vi "TotalAlkalinityTool.vi"() -> ()   [LabVIEW 2010]
uses:
  Misc/HCl_volume_global.vi
panel:
  out "In hold?":bool
  out "Hold Start Time":timestamp
  in  "Tab Control":T1(tab)
  out "Cell Temp (dup)":dbl
  out "Initialized?":bool
  in  "Initialize Instruments":bool
  in  "Run Settings":T2={"Operator"="", "Sample (or CRM) ID"="", "Sample Temp"=0.0, "Salinity"=0.0, "Sample Units"=FALSE, "Sample Size"=0.0, "Operation Mode"=TRUE}
  in  "Data Directory":path
  in  "stop":bool
  in  "Begin Titration":bool
  in  "Configuration":T3={"Alkalinity Calculation Functions"={"HCl Temp Correction Function"="", "Sample Temp Correction Function"="", "Dosimat Correction Function"="", "Cell Temp Correction Function"="", "HCl Density Function"=""}, "Instrument Settings"={"Relay Port"="COM6", "Agilent Port"="COM5", "Dosimat Port"="COM4", "Thermal Coeffients Path"=path ""}, "Titration Settings"={"Hold Time (sec)"=300, "Initial HCl Increment"=0.0, "Target EMF"=0.0, "Agilent Monitoring Refresh Period"=0.0, "Small HCl Increment"=0.0, "Number of Titration Points"=0}, "Other Settings"={"HCl Concentration"=0.0, "HCl Lot ID"=""}, "Electrode Settings"={"Probe ID - Electrode 1 "=0, "Channel - Electrode 1"=0, "Probe ID - Electrode 2"=0, "Channel - Electrode 2"=0}} {"Electrode Settings"."Probe ID - Electrode 2" items=["OLD1", "OLD2", "OV1-106509", "OW1-10628", "OW1-10659"]; "Electrode Settings"."Probe ID - Electrode 1" items=["OLD1", "OLD2", "OV1-106509", "OW1-10628", "OW1-10659"]}
  in  "Save Config":bool
  out "Voltage 2":dbl
  out "Voltage 1":dbl
  out "Titration Pts Left":dbl
  out "Electrode 2 Results":T4 {"k" format="%.5g"; "Final E0" format="%#.5g"; "mse" format="%.2g"}
  out "Electrode 1 Results":T4 {"k" format="%.5g"; "Final E0" format="%#.5g"; "mse" format="%#_3g"}
  out "Titration State":string
  out "Titrating?":bool
  out "Titration EMFs":cluster{"x values":dbl[], "voltages":dbl[]}[](graph)
  out "Voltage Standard Deviation":T5(graph)
  out "Hold Time Remaining":dbl
  out "Burette Temp 2":dbl
  out "Cell Temp":dbl
  out "Acid Temp":dbl
  out "Burette Temp 1":dbl
  out "Room Temp":dbl
  out "HCl Volume (Uncorr)":dbl
  in  "Probe to Follow":bool
  out "E0 Values":cluster{timestamp[], dbl[]}[](graph)
  out "Alakalinity Variance From References":cluster{timestamp[], dbl[]}[](graph)
  in  "Load QC Data":bool
  out "File Error Out":errorcluster
  # "It is important that these settings be correctly set for each run."
  # "y = -0.0003x2 + 1.0021x - 0.003"
  # "Required Inputs"
  # "It is imortant that these settings be correctly set for each run."
  # "These configuration settings are stored in an XML file and can be updated for a specific run and then discarded, but can also be saved by clicking the button to the right.\n\nIf you need to change the instrument port settings, run the config_file_accessor vi in the Misc directory. That iwll let you create a new configuration set."
  # "add new electrode using qc_data_accessor"
  # "This control only works when titration is not actively taking place"
  # "Titration Results"
  # "Temps"
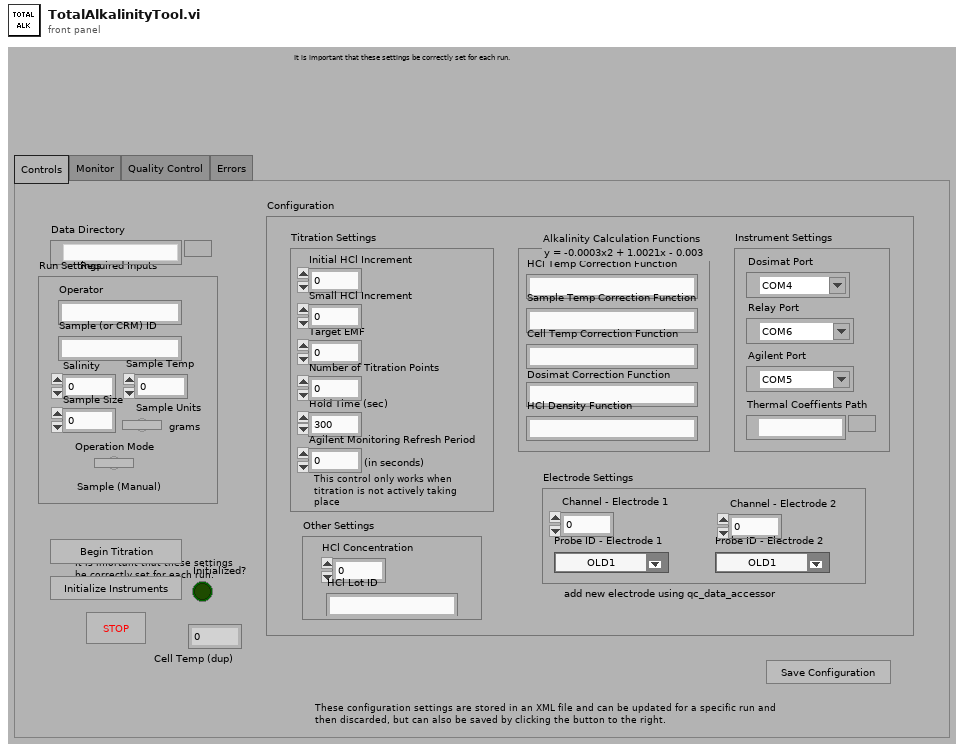
[diagram p1: front panel]
types:
  T1 = enum32{"Controls", "Monitor", "Quality Control", "Errors"}
  T2 = cluster{"Operator":string, "Sample (or CRM) ID":string, "Sample Temp":dbl, "Salinity":dbl, "Sample Units":bool, "Sample Size":dbl, "Operation Mode":bool}
  T3 = cluster{"Alkalinity Calculation Functions":cluster{"HCl Temp Correction Function":string, "Sample Temp Correction Function":string, "Dosimat Correction Function":string, "Cell Temp Correction Function":string, "HCl Density Function":string}, "Instrument Settings":cluster{"Relay Port":refnum<visa-resource-name>, "Agilent Port":refnum<visa-resource-name>, "Dosimat Port":refnum<visa-resource-name>, "Thermal Coeffients Path":path}, "Titration Settings":cluster{"Hold Time (sec)":i16, "Initial HCl Increment":dbl, "Target EMF":dbl, "Agilent Monitoring Refresh Period":dbl, "Small HCl Increment":dbl, "Number of Titration Points":i32}, "Other Settings":cluster{"HCl Concentration":dbl, "HCl Lot ID":string}, "Electrode Settings":cluster{"Probe ID - Electrode 1 ":u16, "Channel - Electrode 1":i32, "Probe ID - Electrode 2":u16, "Channel - Electrode 2":i32}}
  T4 = cluster{"Total Alkalinity":dbl, "mse":dbl, "Final E0":dbl, "k":dbl}
  T5 = cluster{"x values":dbl[], "voltage stddevs":dbl[]}[]
  T6 = cluster{"Time Stamp":timestamp, "Titration Stage":string, "Average Voltage":dbl, "Burette Temp Average":dbl, "Voltage 1":dbl, "Voltage 2":dbl, "Voltage 1 StandDev":dbl, "Voltage 2 StandDev":dbl, "Burette Temp 1":dbl, "Burette Temp 2":dbl, "Cell Temp":dbl, "Acid Temp":dbl, "Room Temp":dbl}[]
  T7 = typedef "LVStringsAndValuesArrayTypeDef.ctl" = cluster{"String":string, "Value":ext}[]
  T8 = cluster{"VISA resource out":refnum<visa-resource-name>, "error out":errorcluster}
  T9 = cluster{"Dosimat Port out":refnum<visa-resource-name>, "Error out":errorcluster}
  T10 = cluster{"Data Flag":string, "Notes":string, "Probe 1 Results":cluster{"Total Alkalinity":dbl, "mse":dbl, "Final E0":dbl, "k":dbl}, "Probe 2 Results":cluster{"Total Alkalinity":dbl, "mse":dbl, "Final E0":dbl, "k":dbl}}
  T11 = cluster{"HCl Temp Correction Function":string, "Sample Temp Correction Function":string, "Dosimat Correction Function":string, "Cell Temp Correction Function":string, "HCl Density Function":string}
  T12 = cluster{"Hold Time (sec)":i16, "Initial HCl Increment":dbl, "Target EMF":dbl, "Agilent Monitoring Refresh Period":dbl, "Small HCl Increment":dbl, "Number of Titration Points":i32}
  T13 = cluster{"HCl Concentration":dbl, "HCl Lot ID":string}
  T14 = cluster{"Relay Port":refnum<visa-resource-name>, "Agilent Port":refnum<visa-resource-name>, "Dosimat Port":refnum<visa-resource-name>, "Thermal Coeffients Path":path}
  T15 = cluster{"Probe ID - Electrode 1 ":u16, "Channel - Electrode 1":i32, "Probe ID - Electrode 2":u16, "Channel - Electrode 2":i32}
  T16 = cluster{"Time":timestamp, "Operator":string, "Flag":string, "CRM ID":string, "HCl Batch ID":string, "CRM Certified Alk":dbl, "Salinity":dbl, "HCl Temp (uncorr)":dbl, "Cell Temp Mean (uncorr)":dbl, "Measured Alk":dbl, "MSE":dbl, "Final E0":dbl, "k":dbl}[]
  T17 = cluster{"Time":timestamp, "Operator":string, "Flag":string, "CRM ID":string, "HCl Batch ID":string, "CRM Certified Alk":dbl, "Salinity":dbl, "HCl Temp (uncorr)":dbl, "Cell Temp Mean (uncorr)":dbl, "Measured Alk":dbl, "MSE":dbl, "Final E0":dbl, "k":dbl}[][]
  T18 = cluster{"Time Stamp":timestamp, "Titration Stage":string, "Average Voltage":dbl, "Burette Temp Average":dbl, "Voltage 1":dbl, "Voltage 2":dbl, "Voltage 1 StandDev":dbl, "Voltage 2 StandDev":dbl, "Burette Temp 1":dbl, "Burette Temp 2":dbl, "Cell Temp":dbl, "Acid Temp":dbl, "Room Temp":dbl}
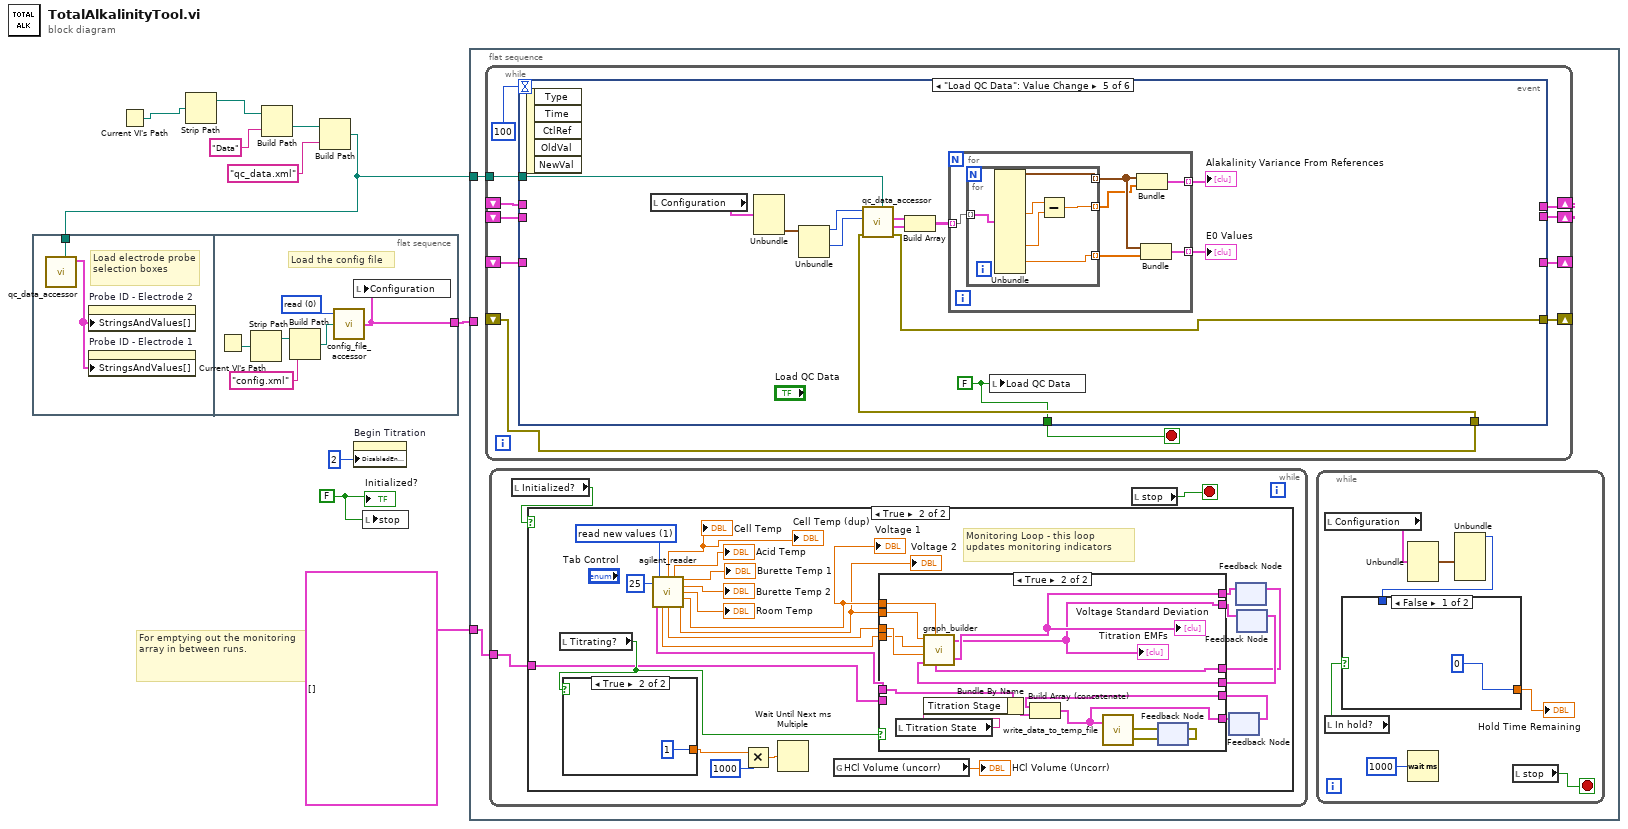
[diagram p0: block diagram]
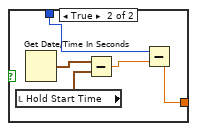
[diagram p2: hidden frame]
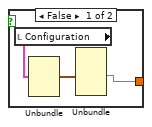
[diagram p4: hidden frame]
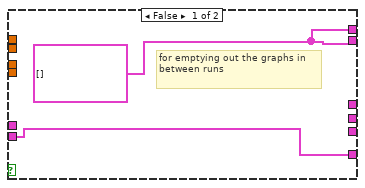
[diagram p5: hidden frame]
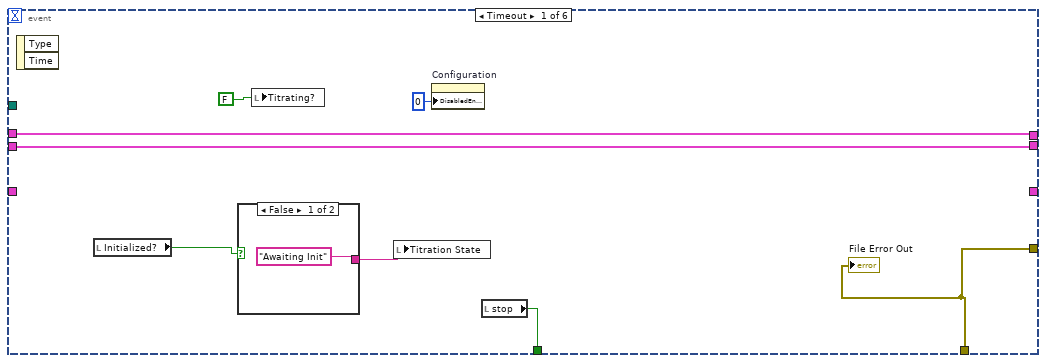
[diagram p6: hidden frame]
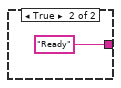
[diagram p7: hidden frame]
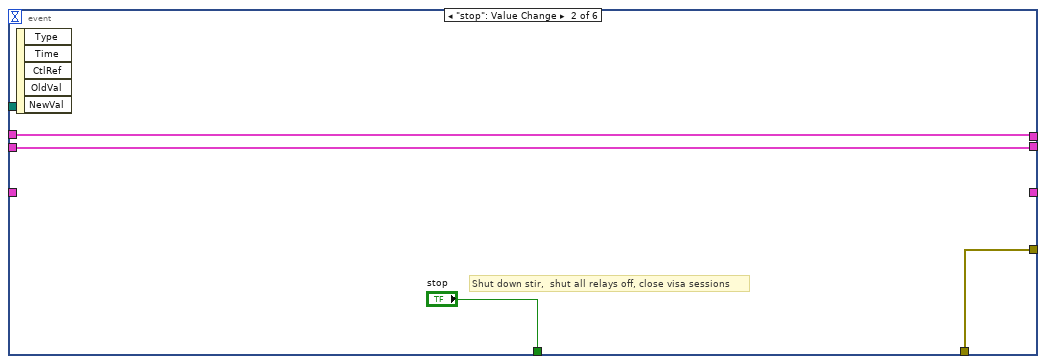
[diagram p8: hidden frame]
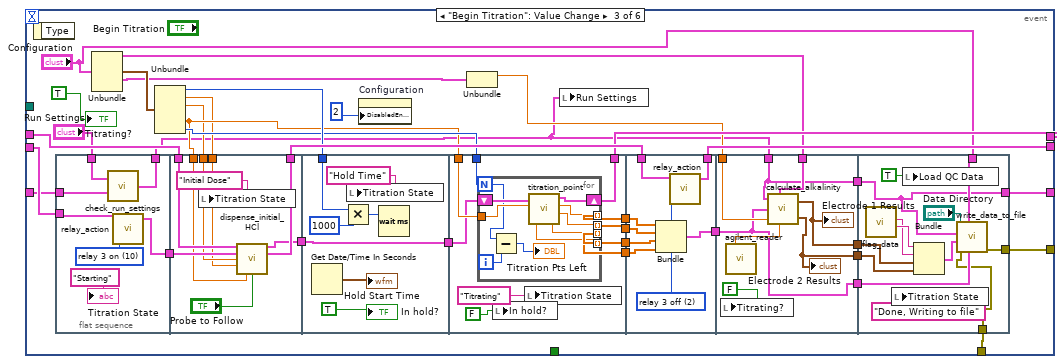
[diagram p9: hidden frame]
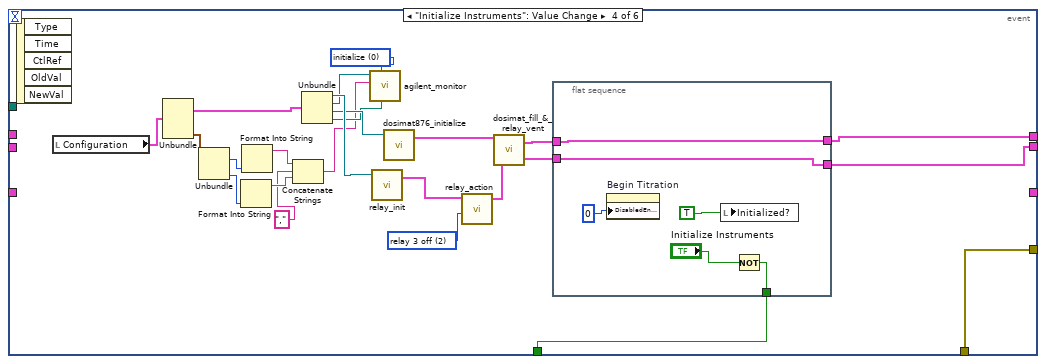
[diagram p10: hidden frame]
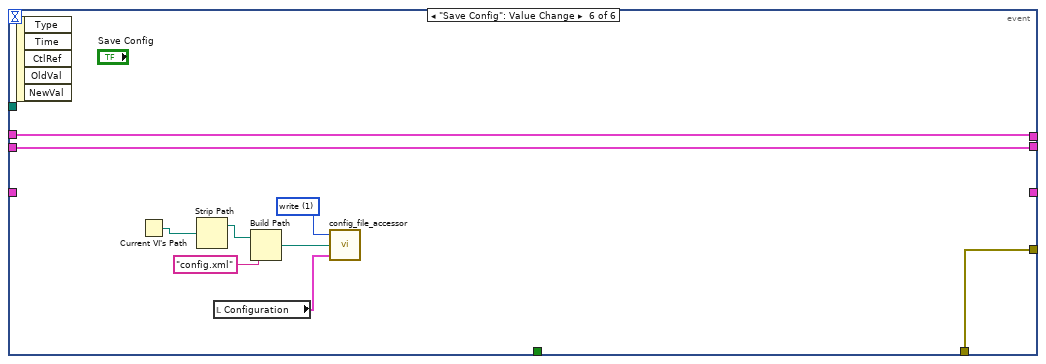
[diagram p11: hidden frame]
diagram:
  w7 = FALSE
  # "For emptying out the monitoring array in between runs."
  n1 = flat-sequence {
    tunnel: w1 -> [w11]
    tunnel: [w13] -> w8
    frame #0 {
      # "Load electrode probe selection boxes"
      n2 = call "qc_data_accessor.vi"("Path"=w11) -> ("Electrode Selection Options"=w12:T7)  [unwired: 7 in, 3 out]
      n3 = property on="Probe ID - Electrode 2" class="Ring (strict)"("StringsAndValues[]"=w12) -> ()  [unwired: 2 in, 2 out]
      n4 = property on="Probe ID - Electrode 1" class="Ring (strict)"("StringsAndValues[]"=w12) -> ()  [unwired: 2 in, 2 out]
    }
    frame #1 {
      w16 = u8 0 items=["read", "write"] ("Action")
      # "Load the config file"
      n5 = Current VI's Path() -> (path=w15:path)
      n6 = Strip Path(path=w15) -> (stripped path=w14:path)  [unwired: 1 out]
      n7 = Build Path(base path=w14, name or relative path="config.xml") -> (appended path=w17:path)
      n8 = call "config_file_accessor.vi"("File Path"=w17, "Action"=w16) -> ("Configuration Out"=w13:T3)  [unwired: 1 in]
      n9 = local write "Configuration"(w13) -> ()
    }
  }
  n10 = Current VI's Path() -> (path=w3:path)
  n11 = Strip Path(path=w3) -> (stripped path=w2:path)  [unwired: 1 out]
  n12 = Build Path(base path=w2, name or relative path="Data") -> (appended path=w4:path)
  n13 = Build Path(base path=w4, name or relative path="qc_data.xml") -> (appended path=w1:path)
  n14 = property on="Begin Titration" class="Bool"("DisabledEnum"=2) -> ()  [unwired: 2 in, 2 out]
  n15 = local write "stop"(w7) -> ()
  n16 = flat-sequence {
    tunnel: T6 [] ("Data Array") -> [w20]
    tunnel: w8 -> [_]
    tunnel: w1 -> [w19]
    frame #0 {
      n17 = while {
        shift-right: [w89] -> _
        shift-left: _ -> [w90]
        shift-right: [w88] -> _
        shift-left: _ -> [w91]
        shift-right: [w86] -> _
        shift-left: _ -> [w85]
        shift-right: [w84] -> _
        shift-left: _ -> [w83]
        tunnel: w19 -> [w82]
        stop <- w92 stop-if-true
        n18 = event shown="[4] \"Load QC Data\": Value Change" {
          selector: _ -> [_ _ _ _ _ _]
          dyn-events: _ -> [_ _ _ _ _ _]
          timeout: 100 -> [_ _ _ _ _ _]
          tunnel: [w93 "stop" _ w237 w247 _] -> w92
          tunnel: w91 -> [w98 w104 w141 _ _ w272]
          tunnel: w90 -> [w99 w105 w140 _ _ w273]
          tunnel: [w99 w105 w136 w225 _ w273] -> w89
          tunnel: [w98 w104 w135 w224 _ w272] -> w88
          tunnel: [w94 w103 w112 w214 w248 w269] -> w86
          tunnel: w85 -> [w94 w103 w111 w214 w249 w269]
          tunnel: [_ _ w110 _ _ _] -> w84
          tunnel: w83 -> [_ _ w108 _ _ _]
          tunnel: w82 -> [_ _ _ _ w244 _]
          event Timeout {
            n19 = event-data() -> ()  [unwired: 1 in, 2 out]
            n20 = local read "Initialized?"() -> (w95:bool)
            n21 = case shown="False" w95 {
              tunnel: ["Awaiting Init" "Ready"] -> w100
              frame False {
              }
              frame True {
              }
            }
            n22 = local write "Titrating?"(FALSE) -> ()
            n23 = local write "Titration State"(w100) -> ()
            n24 = property on="Configuration" class="Clust (strict)"("DisabledEnum"=0) -> ()  [unwired: 2 in, 2 out]
            n25 = local read "stop"() -> (w93:bool)
            "File Error Out" <- w94
          }
          event "stop": Value Change {
            # "Shut down stir,  shut all relays off, close visa sessions"
            n26 = event-data() -> ()  [unwired: 1 in, 5 out]
          }
          event "Begin Titration": Value Change {
            n27 = event-data() -> ()  [unwired: 1 in, 1 out]
            n28 = flat-sequence {
              tunnel: w141 -> [w147]
              tunnel: [w146] -> w139
              tunnel: [w144] -> w107
              tunnel: "Run Settings" -> [w143]
              tunnel: w108 -> [w142]
              tunnel: w140 -> [w157]
              tunnel: w139 -> [w156]
              tunnel: [w155] -> w138
              tunnel: w122 -> [w153]
              tunnel: w121 -> [w152]
              tunnel: w123 -> [w151]
              tunnel: [w150] -> w129
              tunnel: w130 -> [w161]
              tunnel: w129 -> [w158]
              tunnel: [w158] -> w128
              tunnel: w124 -> [w173]
              tunnel: [w172] -> w136
              tunnel: [w171] -> w134
              tunnel: [w170] -> w133
              tunnel: w123 -> [w168]
              tunnel: w128 -> [w167]
              tunnel: [w166] -> w119
              tunnel: [w165] -> w118
              tunnel: w138 -> [w191]
              tunnel: [w190] -> w135
              tunnel: w134 -> [w189]
              tunnel: w133 -> [w188]
              tunnel: [w187] -> w125
              tunnel: w119 -> [w186]
              tunnel: w118 -> [w185]
              tunnel: w132 -> [w194]
              tunnel: w126 -> [w199]
              tunnel: w125 -> [w195]
              tunnel: [w195] -> w120
              tunnel: [w198] -> w117
              tunnel: [w197] -> w116
              tunnel: [w193] -> w113
              tunnel: w107 -> [w193]
              tunnel: w120 -> [w208]
              tunnel: w117 -> [w210]
              tunnel: w116 -> [w209]
              tunnel: "Configuration" -> [w211]
              tunnel: w113 -> [w201]
              tunnel: [w203] -> w112
              tunnel: w111 -> [w202]
              tunnel: [w201] -> w110
              frame #0 {
                w148 = u8 10 items=["relay 1 on"=8, "relay 2 on"=9, "relay 3 on"=10, "relay 4 on"=11, "relay 1 off"=0, "relay 2 off"=1, "relay 3 off"=2, "relay 4 off"=3, "OpenAll"=30, "CloseAll"=29] ("Action 2")
                n29 = call "check_run_settings.vi"("Last Run Settings"=w142, "Current Run Settings"=w143) -> ("New Run Settings"=w144:T2)
                n30 = call "relay_action.vi"("relay session in"=w147, "Action"=w148) -> ("relay session out"=w146:T8)  [unwired: 6 in]
                "Titration State" <- "Starting"
              }
              frame #1 {
                n31 = local write "Titration State"("Initial Dose") -> ()
                n32 = call "dispense_initial_HCl.vi"("Dosimat In"=w157, "relay session in"=w156, "Target EMF"=w153, "Initial HCl Increment"=w152, "Small Increment Size"=w151, "Probe to Follow"="Probe to Follow") -> ("Dosimat Out"=w150:T9, "relay session out"=w155:T8)  [unwired: 8 in]
              }
              frame #2 {
                n33 = Get Date/Time In Seconds() -> (seconds since 1Jan1904=→"Hold Start Time":timestamp)
                n34 = Multiply(x=w161, y=1000) -> (x*y=w160:i32)
                n35 = local write "Titration State"("Hold Time") -> ()
                n36 = Wait (ms)(milliseconds to wait=w160) -> ()  [unwired: 1 out]
                "In hold?" <- TRUE
              }
              frame #3 {
                n37 = for {
                  N: w173 -> [w177]
                  shift-right: [w183] -> w172
                  shift-left: w167 -> [w184]
                  tunnel: [w182] -> w171 mode=indexing
                  tunnel: [w181] -> w170 mode=indexing
                  tunnel: [w180] -> w166 mode=indexing
                  tunnel: w168 -> [w178]
                  tunnel: [w179] -> w165 mode=indexing
                  i -> [w176]
                  n38 = Subtract(x=w177, y=w176) -> (x-y=→"Titration Pts Left":i32)
                  n39 = call "titration_point.vi"("Small HCl incriment"=w178, "Dosimat In"=w184) -> ("EMF 1"=w180:dbl, "Total HCl Volume"=w181:dbl, "Cell Temp"=w182:dbl, "Dosimat Out"=w183:T9, "EMF 2"=w179:dbl)  [unwired: 1 in]
                }
                n40 = local write "In hold?"(FALSE) -> ()
                n41 = local write "Titration State"("Titrating") -> ()
              }
              frame #4 {
                w192 = u8 2 items=["relay 1 on"=8, "relay 2 on"=9, "relay 3 on"=10, "relay 4 on"=11, "relay 1 off"=0, "relay 2 off"=1, "relay 3 off"=2, "relay 4 off"=3, "OpenAll"=30, "CloseAll"=29] ("Action 2")
                n42 = Bundle(w189, w188, w186, w185) -> (w187:cluster{dbl[], dbl[], dbl[], dbl[]})  [unwired: 1 in]
                n43 = call "relay_action.vi"("relay session in"=w191, "Action"=w192) -> ("relay session out"=w190:T8)  [unwired: 6 in]
              }
              frame #5 {
                n44 = local write "Titrating?"(FALSE) -> ()
                n45 = call "agilent_reader.vi"() -> ("Burette Temp Average"=w196:dbl)  [unwired: 4 in, 11 out]
                n46 = call "calculate_alkalinity.vi"("Run Settings"=w193, "Alkalinity Calculation Functions"=w194, "Titration Points"=w195, "HCl Concentration"=w199, "HCl Temp (uncorr)"=w196) -> ("Probe 1 Results"=w198:T4, "Probe 2 Results"=w197:T4)
                "Electrode 1 Results" <- w198
                "Electrode 2 Results" <- w197
              }
              frame #6 {
                n47 = call "flag_data.vi"() -> ("Notes"=w206:string, "Data Flag"=w207:string)  [unwired: 16 in, 2 out]
                n48 = local write "Titration State"("Done, Writing to file") -> ()
                n49 = local write "Load QC Data"(TRUE) -> ()
                n50 = Bundle("Data Flag"=w207, "Notes"=w206, "Probe 1 Results"=w210, "Probe 2 Results"=w209) -> (w205:T10)  [unwired: 1 in]
                n51 = call "write_data_to_file.vi"("Titration Points"=w208, "Configuration"=w211, "error in (no error)"=w202, "Run Data"=w205, "Run Settings"=w201, "Path"="Data Directory") -> ("error out"=w203:errorcluster)  [unwired: 5 in]
              }
            }
            n52 = Unbundle("Configuration") -> ("Alkalinity Calculation Functions"=w132:T11, "Titration Settings"=w131:T12, "Other Settings"=w127:T13)  [unwired: 2 out]
            n53 = Unbundle(w131) -> ("Hold Time (sec)"=w130:i16, "Initial HCl Increment"=w121:dbl, "Target EMF"=w122:dbl, "Small HCl Increment"=w123:dbl, "Number of Titration Points"=w124:i32)  [unwired: 1 out]
            n54 = property on="Configuration" class="Clust (strict)"("DisabledEnum"=2) -> ()  [unwired: 2 in, 2 out]
            n55 = Unbundle(w127) -> ("HCl Concentration"=w126:dbl)  [unwired: 1 out]
            n56 = local write "Run Settings"(w107) -> ()
            "Titrating?" <- TRUE
          }
          event "Initialize Instruments": Value Change {
            w222 = u8 0 items=["initialize", "read"] ("Action")
            w233 = u8 2 items=["relay 1 on"=8, "relay 2 on"=9, "relay 3 on"=10, "relay 4 on"=11, "relay 1 off"=0, "relay 2 off"=1, "relay 3 off"=2, "relay 4 off"=3, "OpenAll"=30, "CloseAll"=29] ("Action 2")
            n57 = event-data() -> ()  [unwired: 1 in, 5 out]
            n58 = local read "Configuration"() -> (w231:T3)
            n59 = Unbundle(w231) -> ("Instrument Settings"=w236:T14, "Electrode Settings"=w221:T15)  [unwired: 3 out]
            n60 = Unbundle(w221) -> ("Channel - Electrode 1"=w220:i32, "Channel - Electrode 2"=w219:i32)  [unwired: 2 out]
            n61 = Format Into String(w219) -> (resulting string=w217:string)  [unwired: 3 in, 1 out]
            n62 = Format Into String(w220) -> (resulting string=w218:string)  [unwired: 3 in, 1 out]
            n63 = Concatenate Strings(w218, ",", w217) -> (w215:string)
            n64 = Unbundle(w236) -> ("Relay Port"=w230:refnum<visa-resource-name>, "Agilent Port"=w227:refnum<visa-resource-name>, "Dosimat Port"=w229:refnum<visa-resource-name>, "Thermal Coeffients Path"=w228:path)
            n65 = call "agilent_monitor.vi"("Thermal Coefficient Path"=w228, "Action"=w222, "voltage channels (csv)"=w215, "Agilent Port In"=w227) -> ()  [unwired: 5 in, 3 out]
            n66 = call "relay_init.vi"("VISA resource in"=w230) -> ("relay session out"=w232:T8)  [unwired: 3 in]
            n67 = call "dosimat876_initialize.vi"("Dosimat Port In"=w229) -> ("Dosimat Out"=w234:T9)  [unwired: 2 in]
            n68 = call "relay_action.vi"("relay session in"=w232, "Action"=w233) -> ("relay session out"=w235:T8)  [unwired: 6 in]
            n69 = call "dosimat_fill_&_relay_vent.vi"("relay session in"=w235, "Dosimat In"=w234) -> ("relay session out"=w223:T8, "Dosimat Out"=w226:T9)
            n70 = flat-sequence {
              tunnel: [w243] -> w237
              tunnel: [w239] -> w225
              tunnel: w226 -> [w239]
              tunnel: [w238] -> w224
              tunnel: w223 -> [w238]
              frame #0 {
                n71 = property on="Begin Titration" class="Bool"("DisabledEnum"=0) -> ()  [unwired: 2 in, 2 out]
                n72 = local write "Initialized?"(TRUE) -> ()
                n73 = Not(x="Initialize Instruments") -> (.not. x?=w243:bool)
              }
            }
          }
          event "Load QC Data": Value Change {
            w247 = FALSE
            n74 = event-data() -> ()  [unwired: 1 in, 5 out]
            n75 = local read "Configuration"() -> (w256:T3)
            n76 = Unbundle(w256) -> ("Electrode Settings"=w255:T15)  [unwired: 4 out]
            n77 = Unbundle(w255) -> ("Probe ID - Electrode 1"=w254:u16, "Probe ID - Electrode 2"=w253:u16)  [unwired: 2 out]
            n78 = call "qc_data_accessor.vi"("Path"=w244, "error in (no error)"=w249, "Electrode 2 Index"=w253, "Electrode 1 Index"=w254) -> ("error out"=w248:errorcluster, "CRM History - Electrode 2"=w251:T16, "CRM History - Electrode 1"=w252:T16)  [unwired: 4 in, 1 out]
            n79 = Build Array(w252, w251) -> (w250:T17)
            n80 = for {
              tunnel: w250 -> [w262] mode=indexing
              tunnel: [w258] -> w245 mode=indexing
              tunnel: [w257] -> w246 mode=indexing
              n81 = for {
                tunnel: w262 -> [w268] mode=indexing
                tunnel: [w267] -> w261 mode=indexing
                tunnel: [w266] -> w260 mode=indexing
                tunnel: [w265] -> w259 mode=indexing
                n82 = Unbundle(w268) -> ("Time"=w267:timestamp, "CRM Certified Alk"=w264:dbl, "Measured Alk"=w263:dbl, "Final E0"=w265:dbl)  [unwired: 9 out]
                n83 = Subtract(x=w264, y=w263) -> (x-y=w266:dbl)
              }
              n84 = Bundle(w261, w260) -> (w258:cluster{timestamp[], dbl[]})  [unwired: 1 in]
              n85 = Bundle(w261, w259) -> (w257:cluster{timestamp[], dbl[]})  [unwired: 1 in]
            }
            "Alakalinity Variance From References" <- w245
            "E0 Values" <- w246
            n86 = local write "Load QC Data"(w247) -> ()
          }
          event "Save Config": Value Change {
            w275 = u8 1 items=["read", "write"] ("Action")
            n87 = event-data() -> ()  [unwired: 1 in, 5 out]
            n88 = Current VI's Path() -> (path=w271:path)
            n89 = Strip Path(path=w271) -> (stripped path=w270:path)  [unwired: 1 out]
            n90 = local read "Configuration"() -> (w274:T3)
            n91 = Build Path(base path=w270, name or relative path="config.xml") -> (appended path=w276:path)
            n92 = call "config_file_accessor.vi"("Configuration In"=w274, "File Path"=w276, "Action"=w275) -> ()  [unwired: 1 out]
          }
        }
      }
      n93 = while {
        tunnel: w20 -> [w36]
        stop <- w34 stop-if-true
        n94 = local read "Initialized?"() -> (w35:bool)
        n95 = case shown="True" w35 {
          tunnel: w36 -> [_ w40]
          frame False {
          }
          frame True {
            w55 = u8 1 items=["read new values"=1, "read last values "=2] ("Action")
            # "Monitoring Loop - this loop updates monitoring indicators"
            n96 = local read "Titrating?"() -> (w43:bool)
            n97 = case shown="True" w43 {
              tunnel: [w61 1] -> w44
              frame False {
                n98 = local read "Configuration"() -> (w63:T3)
                n99 = Unbundle(w63) -> ("Titration Settings"=w62:T12)  [unwired: 4 out]
                n100 = Unbundle(w62) -> ("Agilent Monitoring Refresh Period"=w61:dbl)  [unwired: 5 out]
              }
              frame True {
              }
            }
            n101 = call "agilent_reader.vi"("Action"=w55, "Voltage Readings"=25) -> ("Cell Temp"=→"Cell Temp" →"Cell Temp (dup)":dbl, "Acid Temp"=→"Acid Temp":dbl, "Burette Temp 1"=→"Burette Temp 1":dbl, "Burette Temp 2"=→"Burette Temp 2":dbl, "Room Temp"=→"Room Temp":dbl, "Voltage 1"=w39:dbl, "Data Cluster"=w45:T18, "Voltage 1 StandDev"=w51:dbl, "Voltage 2 StandDev"=w52:dbl, "Voltage 2"=w38:dbl)  [unwired: 2 in, 2 out]
            "Voltage 2" <- w38
            "Voltage 1" <- w39
            n102 = Multiply(x=w44, y=1000) -> (x*y=w60:dbl)
            n103 = Wait Until Next ms Multiple(millisecond multiple=w60) -> ()  [unwired: 1 out]
            n104 = global read "HCl_volume_global.vi" "HCl Volume (uncorr)"() -> (→"HCl Volume (Uncorr)":dbl)
            n105 = feedback #1() -> (w41:T6)  [unwired: 1 in]
            n106 = feedback #2() -> (w46:T5)  [unwired: 1 in]
            n107 = feedback #3() -> (w47:cluster{"x values":dbl[], "voltages":dbl[]}[])  [unwired: 1 in]
            n108 = case shown="True" w43 {
              tunnel: w39 -> [_ w81]
              tunnel: w38 -> [_ w80]
              tunnel: w52 -> [_ w68]
              tunnel: w51 -> [_ w67]
              tunnel: w45 -> [_ w79]
              tunnel: [w65 w74] -> w49
              tunnel: [w65 w73] -> w48
              tunnel: w47 -> [_ w72]
              tunnel: w46 -> [_ w71]
              tunnel: [w66 w70] -> w42
              tunnel: w41 -> [_ w69]
              tunnel: w40 -> [w66 _]
              frame False {
                w65 = cluster{"x values":dbl[], "voltages":dbl[]}[] [] ("Voltage Graph in")
                # "for emptying out the graphs in between runs"
              }
              frame True {
                n109 = local read "Titration State"() -> (w78:string)
                n110 = call "graph_builder.vi"("Voltage StdDev Graph in"=w71, "Voltage 1"=w81, "Voltage Graph in"=w72, "Voltage StdDev 2"=w68, "Voltage StdDev 1"=w67, "Voltage 2"=w80) -> ("Voltage StdDev Graph out"=w74:T5, "Voltage Graph out"=w73:cluster{"x values":dbl[], "voltages":dbl[]}[])
                "Titration EMFs" <- w73
                "Voltage Standard Deviation" <- w74
                n111 = Bundle By Name(cluster=w79, "Titration Stage"=w78) -> (w77:T18)
                n112 = Build Array (concatenate)(w69, w77) -> (w70:T6)
                n113 = feedback #4() -> (w75:errorcluster)  [unwired: 1 in]
                n114 = call "write_data_to_temp_file.vi"("error in (no error)"=w75, "Data Array"=w70) -> ("error out"=w76:errorcluster)  [unwired: 1 in]
                n115 = feedback-in #4(w76) -> ()
              }
            }
            n116 = feedback-in #1(w42) -> ()
            n117 = feedback-in #2(w49) -> ()
            n118 = feedback-in #3(w48) -> ()
          }
        }
        n119 = local read "stop"() -> (w34:bool)
      }
      n120 = while {
        stop <- w22 stop-if-true
        n121 = local read "Configuration"() -> (w24:T3)
        n122 = local read "In hold?"() -> (w27:bool)
        n123 = Unbundle(w24) -> ("Titration Settings"=w25:T12)  [unwired: 4 out]
        n124 = Wait (ms)(milliseconds to wait=1000) -> ()  [unwired: 1 out]
        n125 = Unbundle(w25) -> ("Hold Time (sec)"=w23:i16)  [unwired: 5 out]
        n126 = case shown="False" w27 {
          tunnel: [0 w30] -> w26
          tunnel: w23 -> [_ w29]
          frame False {
          }
          frame True {
            n127 = local read "Hold Start Time"() -> (w32:timestamp)
            n128 = Get Date/Time In Seconds() -> (seconds since 1Jan1904=w33:timestamp)
            n129 = Subtract(x=w33, y=w32) -> (x-y=w31:dbl)
            n130 = Subtract(x=w29, y=w31) -> (x-y=w30:dbl)
          }
        }
        "Hold Time Remaining" <- w26
        n131 = local read "stop"() -> (w22:bool)
      }
    }
  }
  "Initialized?" <- w7
